vi "Switch_ReadProtocol.vi"(8 "错误输入（无错误）":errorcluster, 9 "Old通道2":bool, 10 "Old通道1":bool, 11 "COM":refnum<visa-resource-name>) -> (0 "错误输出":errorcluster, 1 "通道2":bool, 2 "通道1":bool, 3 "COM Out":refnum<visa-resource-name>)   [LabVIEW 2018, in "Switch.lvlib"]
uses:
  Switch.lvlib
  <vilib>/Instr/_visa.llb/VISA Flush IO Buffer Mask.ctl
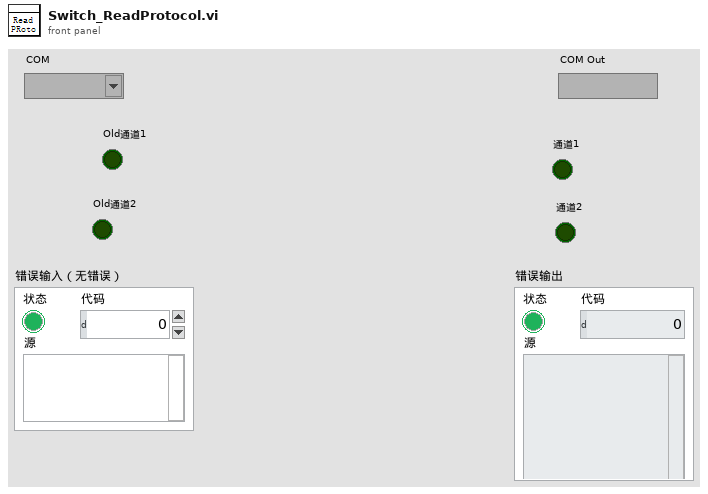
[diagram p1: front panel]
types:
  T1 = typedef "VISA Flush IO Buffer Mask.ctl" = u16
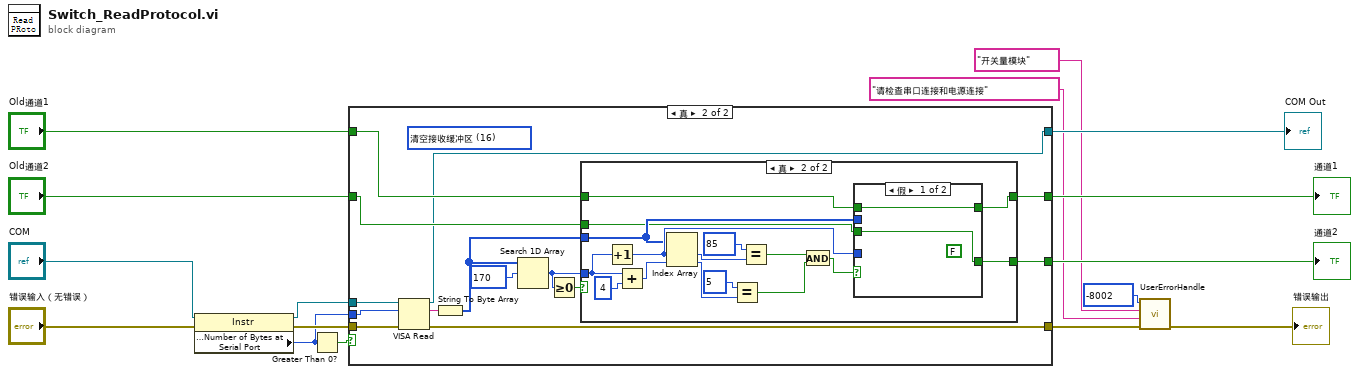
[diagram p0: block diagram]
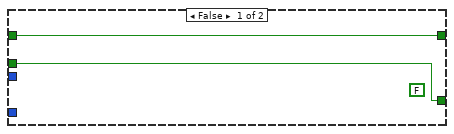
[diagram p3: hidden frame]
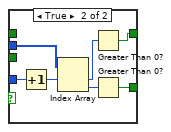
[diagram p4: hidden frame]
diagram:
  n1 = property class="Instr"(reference="COM", error in="错误输入（无错误）") -> (reference out=w15:refnum<visa-resource-name>, error out=w13:errorcluster, "Serial Settings:Number of Bytes at Serial Port"=w10:u32)
  n2 = Greater Than 0?(x=w10) -> (x > 0?=w11:bool)
  n3 = case shown="真" w11 {
    tunnel: w15 -> [w20 w34]
    tunnel: w10 -> [_ w33]
    tunnel: w13 -> [w19 w31]
    tunnel: [w19 w21] -> w2
    tunnel: [w20 w22] -> w12
    tunnel: [w18 w26] -> w9
    tunnel: [w17 w25] -> w8
    tunnel: "Old通道1" -> [w18 w24]
    tunnel: "Old通道2" -> [w17 w23]
    frame False {
    }
    frame True {
      (unwired) T1 16 items=["清空接收缓冲区"=16, "向设备写入传输缓冲区"=32, "清空接收缓冲区（无I/O）"=64, "清空传输缓冲区"=128] ("Mask")
      n4 = VISA Read(VISA resource name=w34, byte count=w33, error in (no error)=w31) -> (VISA resource name out=w22:refnum<visa-resource-name>, read buffer=w32:string, error out=w21:errorcluster)  [unwired: 1 out]
      n5 = String To Byte Array(string=w32) -> (unsigned byte array=w27:u8[])
      n6 = Search 1D Array(1D array=w27, element=u8 170 ("元素")) -> (index of element=w28:i32)  [unwired: 1 in]
      n7 = Greater Or Equal To 0?(x=w28) -> (x >= 0?=w29:bool)
      n8 = case shown="真" w29 {
        tunnel: w28 -> [_ w48]
        tunnel: w27 -> [_ w49]
        tunnel: [w36 w40] -> w26
        tunnel: [w35 w39] -> w25
        tunnel: w24 -> [w36 w38]
        tunnel: w23 -> [w35 w37]
        frame False {
          (unwired) FALSE
        }
        frame True {
          n9 = Increment(x=w48) -> (x+1=w50:i32)
          n10 = Add(x=w48, y=4) -> (x+y=w46:i32)
          n11 = Index Array(array=w49, index #1=w50, index #2=w46) -> (element #1=w51:u8, element #2=w45:u8)
          n12 = Equal?(x=u8 5 ("元素"), y=w45) -> (x = y?=w43:bool)
          n13 = Equal?(x=u8 85 ("元素"), y=w51) -> (x = y?=w42:bool)
          n14 = And(x=w42, y=w43) -> (x .and. y?=w41:bool)
          n15 = case shown="假" w41 {
            tunnel: w49 -> [_ w61]
            tunnel: w50 -> [_ w60]
            tunnel: [w54 w56] -> w40
            tunnel: [w53 w55] -> w39
            tunnel: w38 -> [w54 _]
            tunnel: w37 -> [w53 _]
            frame False {
              (unwired) FALSE
            }
            frame True {
              n16 = Increment(x=w60) -> (x+1=w59:i32)
              n17 = Index Array(array=w61, index #1=w59) -> (element #1=w58:u8, element #2=w57:u8)  [unwired: 1 in]
              n18 = Greater Than 0?(x=w58) -> (x > 0?=w56:bool)
              n19 = Greater Than 0?(x=w57) -> (x > 0?=w55:bool)
            }
          }
        }
      }
    }
  }
  "COM Out" <- w12
  "通道1" <- w9
  "通道2" <- w8
  n20 = call "UserErrorHandle.vi"("错误输入"=w2, "错误解释"="请检查串口连接和电源连接", "错误源"="开关量模块", "错误编号"=-8002) -> ("错误输出"=→"错误输出":errorcluster)  [unwired: 7 in]
